vi "Reset_Lockout.vi"(4 "error in (no error)":errorcluster, 5 "Boiler Simulation Controls":refnum<vi>, 6 "Boiler Controls":refnum<vi>, 7 "Data":T1) -> (0 "error out":errorcluster, 3 "State Out":T2)   [LabVIEW 2023]
uses:
  Controls/State.ctl
  Controls/DataCluster.ctl
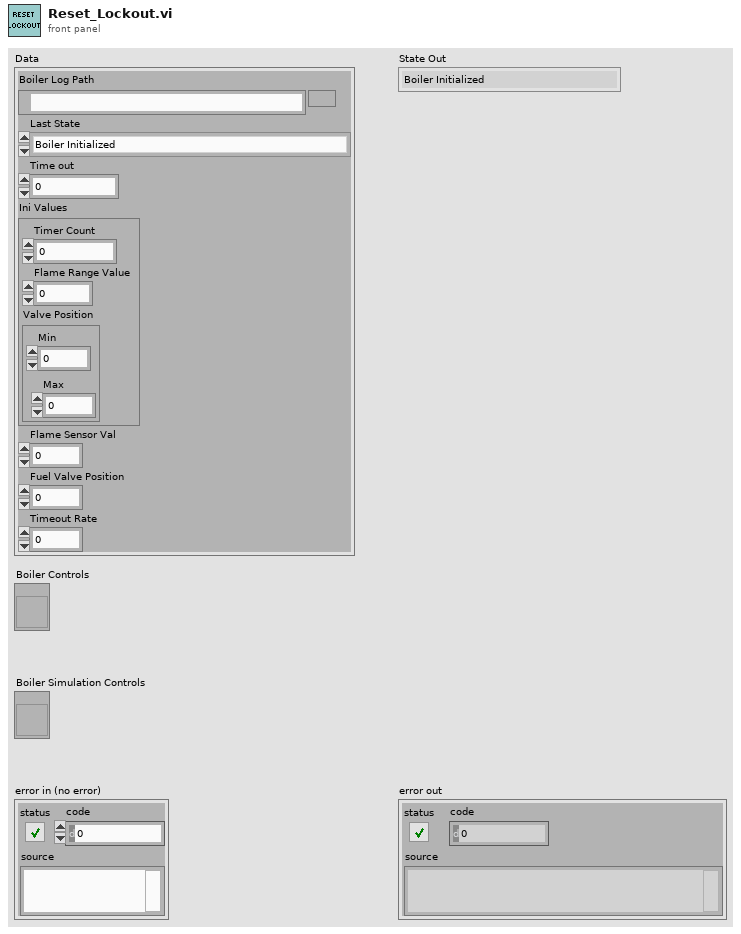
[diagram p1: front panel]
types:
  T1 = typedef "DataCluster.ctl" = cluster{"Boiler Log Path":path, "Last State":T2, "Time out":i32, "Ini Values":cluster{"Timer Count":dbl, "Flame Range Value":dbl, "Valve Position ":cluster{"Min":dbl, "Max":dbl}}, "Flame Sensor Val":dbl, "Fuel Valve Position":dbl, "Timeout Rate":i32}
  T2 = typedef "State.ctl" = enum16{"Boiler Initialized", "Boiler Ready", "Start Pre-Purge", "Pre-Purge Complete", "Pilot On", "Pilot Proved", "Force Draft Fan ON", "Boiler Running", "Start Shutdown Purge", "Shutdown Purge Complete", "Wait for Something"}
  T3 = typedef "Boiler Controls.ctl" = cluster{"Boiler Reset":bool, "Start Sequence":bool, "Pilot":bool, "Shutdown":bool, "Fuel Valve Position":dbl}
  T4 = typedef "Boiler Simulation Controls.ctl" = cluster{"Flame Sensor Value (%)":dbl, "Run Interlock":bool, "Forced Draft Fan":bool}
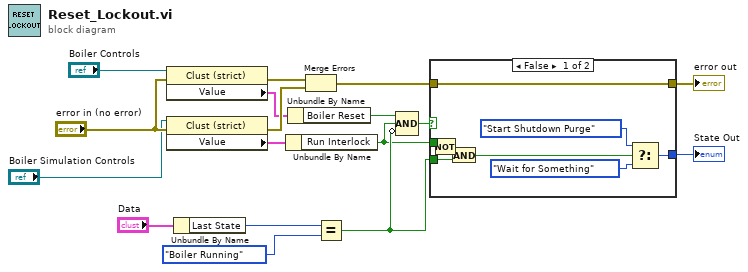
[diagram p0: block diagram]
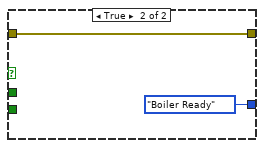
[diagram p2: hidden frame]
diagram:
  n1 = property class="Clust (strict)"(reference="Boiler Controls", error in="error in (no error)") -> (error out=w15:errorcluster, "Value"=w11:T3)  [unwired: 1 out]
  n2 = property class="Clust (strict)"(reference="Boiler Simulation Controls", error in="error in (no error)") -> (error out=w16:errorcluster, "Value"=w13:T4)  [unwired: 1 out]
  n3 = Unbundle By Name("Data") -> ("Last State"=w4:T2)
  n4 = Unbundle By Name(w13) -> ("Run Interlock"=w1:bool)
  n5 = Unbundle By Name(w11) -> ("Boiler Reset"=w6:bool)
  n6 = Merge Errors(w15, w16) -> (w8:errorcluster)
  n7 = Equal?(x=w4, y=State."Boiler Running") -> (x = y?=w2:bool)
  n8 = Compound Arithmetic op=AND(w6, w1, invert w2) -> (w17:bool)
  n9 = case shown="False" w17 {
    tunnel: [w19 State."Boiler Ready"] -> w9
    tunnel: w8 -> [w25 w27]
    tunnel: [w25 w27] -> w7
    tunnel: w2 -> [w24 _]
    tunnel: w1 -> [w23 _]
    frame False {
      n10 = Not(x=w23) -> (.not. x?=w18:bool)
      n11 = And(x=w18, y=w24) -> (x .and. y?=w22:bool)
      n12 = Select(t=State."Start Shutdown Purge", s=w22, f=State."Wait for Something") -> (s? t:f=w19:T2)
    }
    frame True {
    }
  }
  "error out" <- w7
  "State Out" <- w9
